vi "Live Display and capture_3.vi"() -> ()   [LabVIEW 2020]
doc: "The Acquire Every Image (Optimized Performance) example shows the basics of using a ring acquisition. There are some camera restrictions to using this mode that are described in more detail in the block diagram of the VI, but it is recommended to use this method for performance-critical applications when possible."
uses:
  <vilib>/vision/driver/IMAQdx.llb/IMAQdx Acquisition Mode.ctl
  Camera Server/Globals/CamServer global.vi
  <vilib>/vision/driver/NI_Vision_Acquisition_Software.lvlib
  <resource>/objmgr/imaqdx.rc
panel:
  out "Name 3":string
  out "Name 2":string
  out "Name 1":string
  out "Image 3":T1(plugin-control)
  out "Image 2":T1(plugin-control)
  out "error out":errorcluster
  out "Image count":i32
  out "Image 1":T1(plugin-control)
  in  "Stop":bool
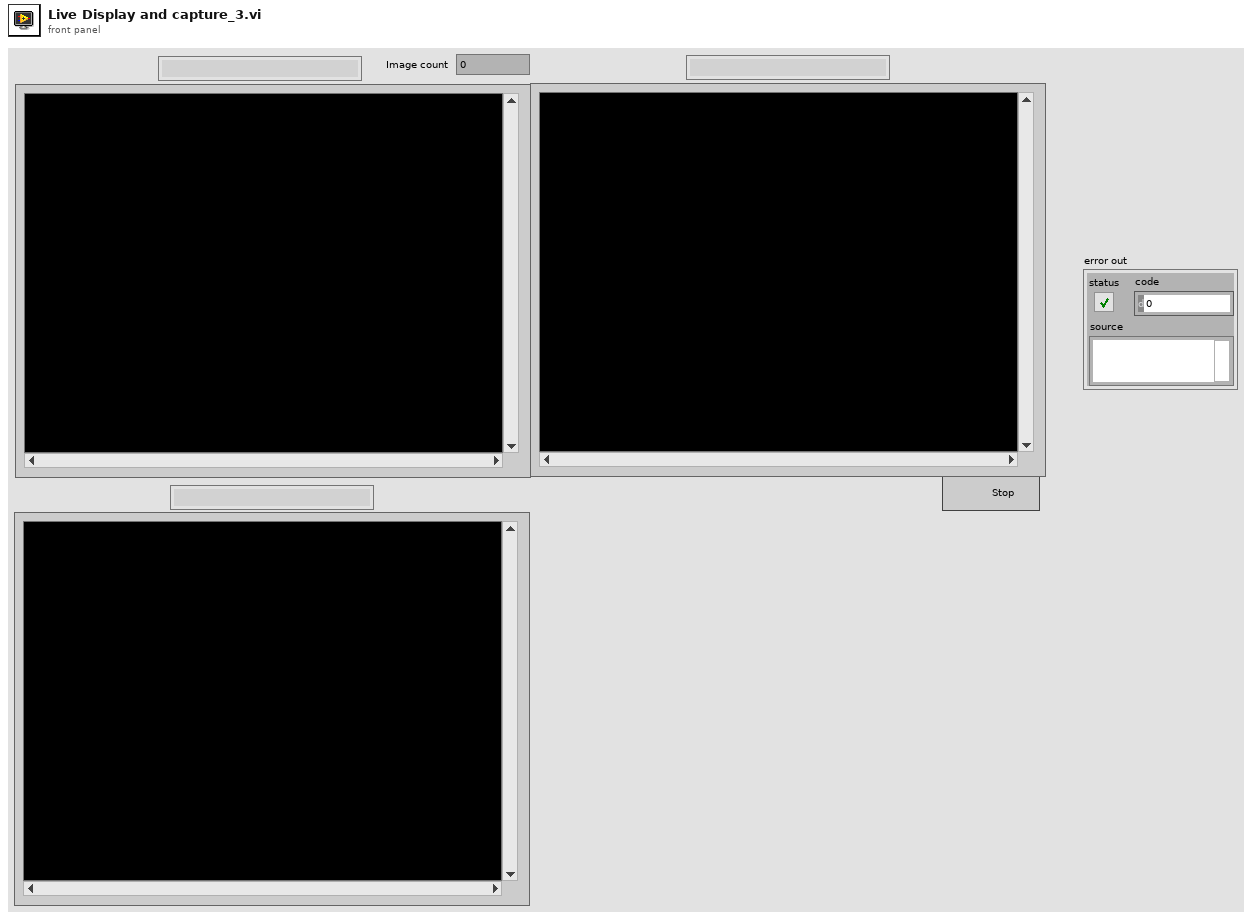
[diagram p1: front panel]
types:
  T1 = typedef "IMAQ Image.ctl" = refnum<image>
  T2 = typedef "NI_Vision_Acquisition_Software.lvlib/IMAQdx Acquisition Mode.ctl" = enum32{"One Shot", "Continuous"}
  T3 = typedef "Camera enum.ctl" = string
  T4 = typedef "IMAQdx.ctl" = refnum<k21>
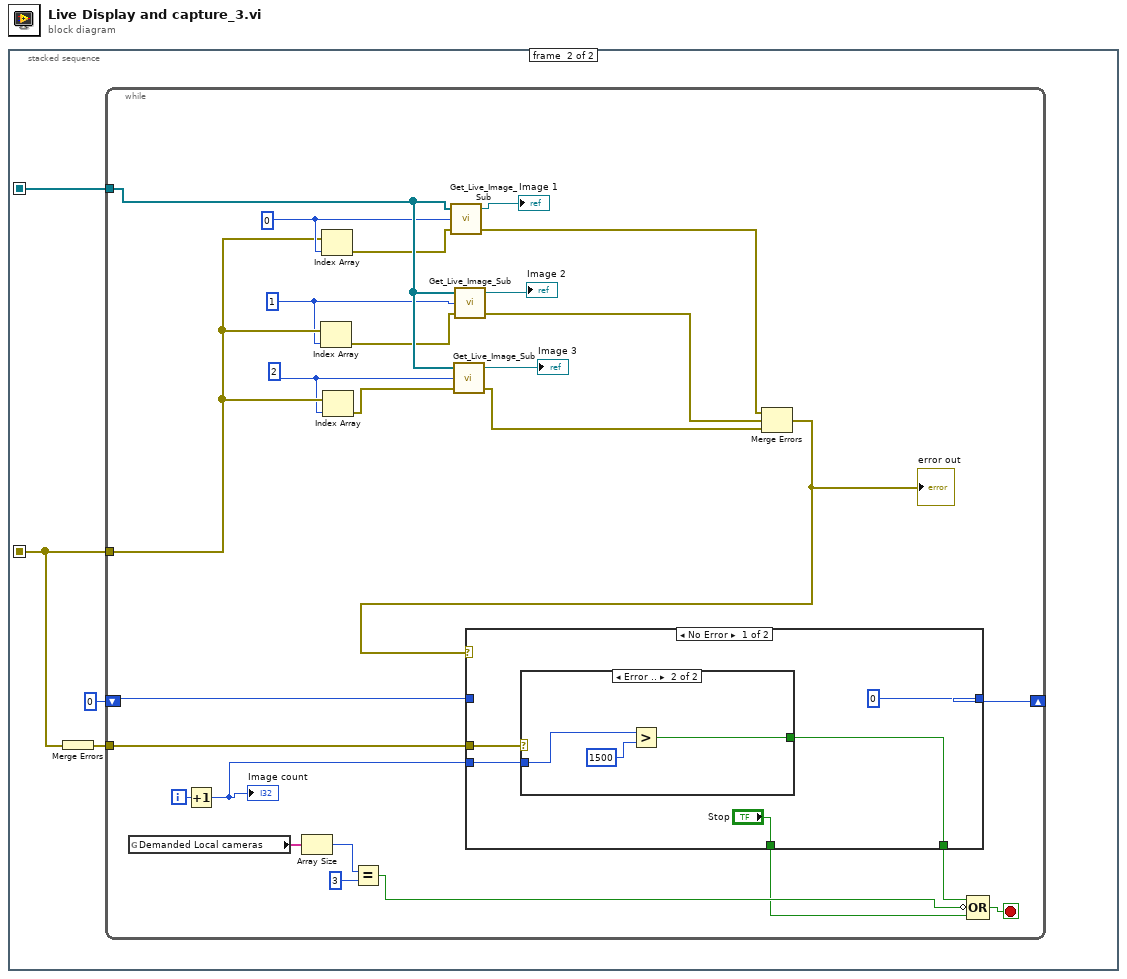
[diagram p0: block diagram]
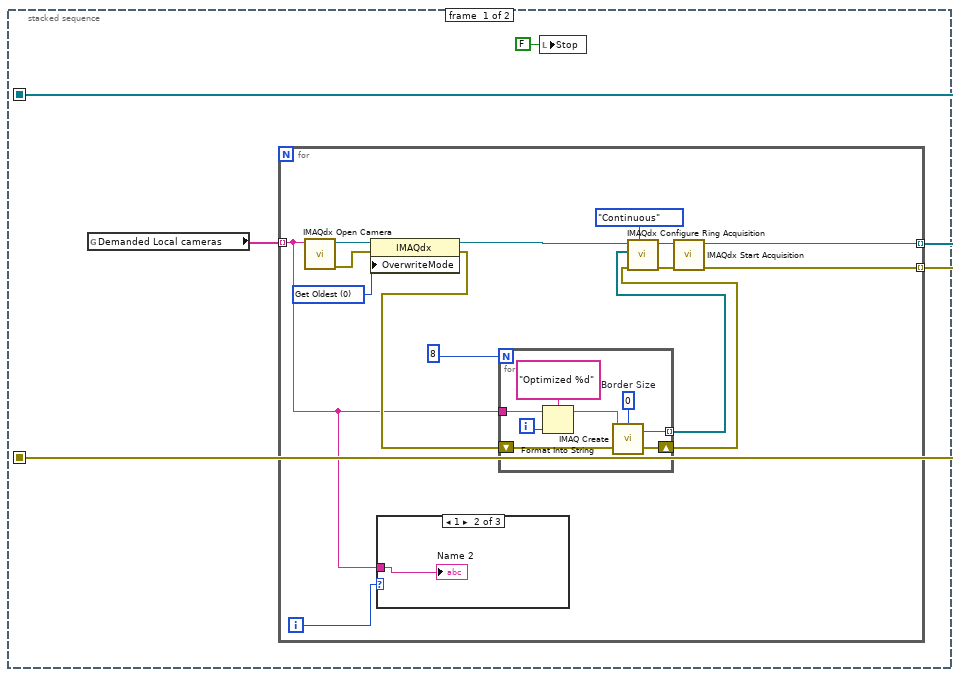
[diagram p2: hidden frame]
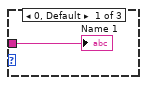
[diagram p3: hidden frame]
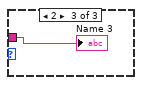
[diagram p4: hidden frame]
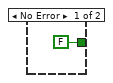
[diagram p5: hidden frame]
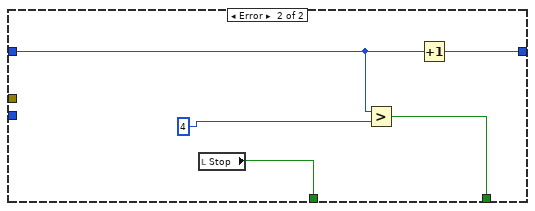
[diagram p6: hidden frame]
diagram:
  n1 = stacked-sequence {
    seq-local: [w4 _] -> [_ w34]
    seq-local: [w3 _] -> [_ w32]
    frame #0 {
      n2 = global read "CamServer global.vi" "Demanded Local cameras"() -> (w2:T3[])
      n3 = for {
        tunnel: w2 -> [w5] mode=indexing
        tunnel: [w13] -> w4 mode=indexing
        tunnel: [w12] -> w3 mode=indexing
        i -> [w6]
        w7 = u32 0 items=["Get Oldest"=0, "Fail"=2, "Get Newest"=3] ("OverwriteMode")
        n4 = call <vilib>:"IMAQdx Open Camera.vi"("Session In"=w5) -> ("error out"=w19:errorcluster, "Session Out"=w18:T4)  [unwired: 2 in, 7 out]
        n5 = property class="IMAQdx"(reference=w18, error in=w19, "OverwriteMode"=w7) -> (reference out=w14:T4, error out=w11:errorcluster)
        n6 = case shown="1" w6 {
          tunnel: w5 -> [w20 w21 w22]
          frame 0, Default {
            "Name 1" <- w20
          }
          frame 1 {
            "Name 2" <- w21
          }
          frame 2 {
            "Name 3" <- w22
          }
        }
        n7 = for {
          N: 8 ("Number of Images") -> [_]
          tunnel: [w29] -> w9 mode=indexing
          shift-right: [w28] -> w10
          shift-left: w11 -> [w30]
          tunnel: w5 -> [w23]
          i -> [w27]
          w24 = 0  # Border Size
          n8 = Format Into String(format string="Optimized %d" ("Image Name"), initial string=w23, w27) -> (resulting string=w26:string)  [unwired: 1 in, 1 out]
          n9 = call "IMAQ Create"("Border Size"=w24, "Image Name"=w26, "error in (no error)"=w30) -> ("New Image"=w29:T1, "error out"=w28:errorcluster)  [unwired: 1 in, 1 out]
        }
        n10 = call <vilib>:"IMAQdx Configure Ring Acquisition.vi"("Mode"=IMAQdx_Acquisition_Mode."Continuous" ("Continuous?"), "error in"=w10, "Images"=w9, "Session In"=w14) -> ("error out"=w16:errorcluster, "Session Out"=w15:T4)  [unwired: 5 in, 1 out]
        n11 = call <vilib>:"IMAQdx Start Acquisition.vi"("error in"=w16, "Session In"=w15) -> ("error out"=w12:errorcluster, "Session Out"=w13:T4)  [unwired: 8 out]
      }
      n12 = local write "Stop"(FALSE ("Stop")) -> ()
    }
    frame #1 {
      n13 = Merge Errors(w32) -> (w31:errorcluster)
      n14 = while {
        tunnel: w34 -> [w55]
        tunnel: w32 -> [w42]
        shift-right: [w47] -> _
        shift-left: 0 -> [w46]
        tunnel: w31 -> [w37]
        i -> [w60]
        stop <- w61 stop-if-true
        w40 = 2 ("y")
        w41 = 1 ("y")
        w43 = 0 ("y")
        n15 = global read "CamServer global.vi" "Demanded Local cameras"() -> (w59:T3[])
        n16 = Increment(x=w60) -> (x+1=w36:i32)
        "Image count" <- w36
        n17 = Array Size(array=w59) -> (size(s)=w58:i32)
        n18 = Index Array(array=w42, index=w41) -> (element=w38:errorcluster)
        n19 = Index Array(array=w42, index=w43) -> (element=w44:errorcluster)
        n20 = Index Array(array=w42, index=w40) -> (element=w39:errorcluster)
        n21 = Equal?(x=w58, y=3) -> (x = y?=w57:bool)
        n22 = call "Get_Live_Image_Sub.vi"("error in"=w44, "index"=w43, "Session Array"=w55) -> ("error out"=w54:errorcluster, "Image"=→"Image 1":T1)  [unwired: 1 in]
        n23 = call "Get_Live_Image_Sub.vi"("error in"=w39, "index"=w40, "Session Array"=w55) -> ("error out"=w52:errorcluster, "Image"=→"Image 3":T1)  [unwired: 1 in]
        n24 = call "Get_Live_Image_Sub.vi"("error in"=w38, "index"=w41, "Session Array"=w55) -> ("error out"=w53:errorcluster, "Image"=→"Image 2":T1)  [unwired: 1 in]
        n25 = Merge Errors(w54, w53, w52) -> (w48:errorcluster)
        "error out" <- w48
        n26 = case shown="No Error" w48 {
          tunnel: [0 w75] -> w47
          tunnel: w46 -> [_ w74]
          tunnel: [w63 w73] -> w45
          tunnel: w37 -> [w65 _]
          tunnel: w36 -> [w64 _]
          tunnel: ["Stop" w71] -> w35
          frame No Error {
            n27 = case shown="Error .." w65 {
              tunnel: w64 -> [_ w69]
              tunnel: [FALSE w68] -> w63
              frame No Error {
              }
              frame Error {
                n28 = Greater?(x=w69, y=1500) -> (0:w68:bool)
              }
            }
          }
          frame Error {
            n29 = local read "Stop"() -> (w71:bool)
            n30 = Greater?(x=w74, y=4) -> (0:w73:bool)
            n31 = Increment(x=w74) -> (x+1=w75:i32)
          }
        }
        n32 = Compound Arithmetic op=OR(w45, invert w57, w35) -> (w61:bool)
      }
    }
  }
